vi "_TangoExtractArchivedData.vi"(2 "error in":errorcluster, 3 "db_extractor_dev_name":string, 4 "sampling":string, 5 "to_date":string, 6 "from_date":string, 7 "archived_attr_name":string) -> (0 "error out":errorcluster, 1 "attr values":T1(array[cluster]))   [LabVIEW 2014, in "tango.lvlib"]
uses:
  tango.lvlib
  Private VIs/Commands/Insertors/fromDevVarStringArray.vi
  Private VIs/Commands/Extractors/toDevVarLongStringArray.vi
  Private VIs/Commands/Insertors/fromDevString.vi
  tango_binding.so
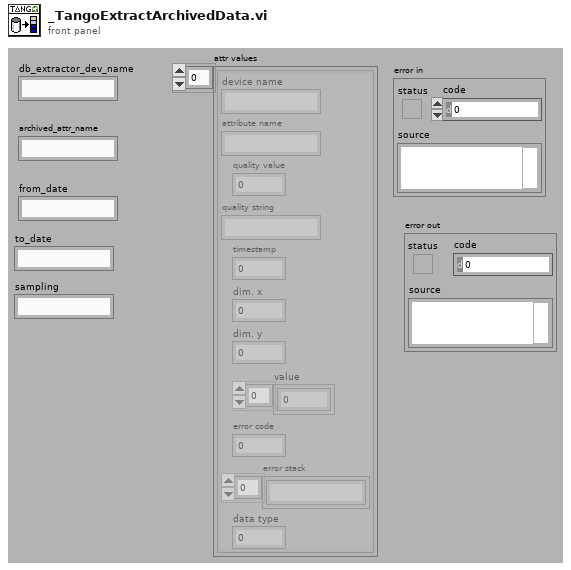
[diagram p1: front panel]
types:
  T1 = cluster{"device name":string, "attribute name":string, "quality value":i16, "quality string":string, "timestamp":dbl, "dim. x":i32, "dim. y":i32, "value":u8[], "error code":i32, "error stack":string[], "data type":u16}[]
  T2 = cluster{"device name":string, "attribute name":string, "quality value":i16, "quality string":string, "timestamp":dbl, "dim. x":i32, "dim. y":i32, "value":u8[], "error code":i32, "error stack":string[], "data type":u16}
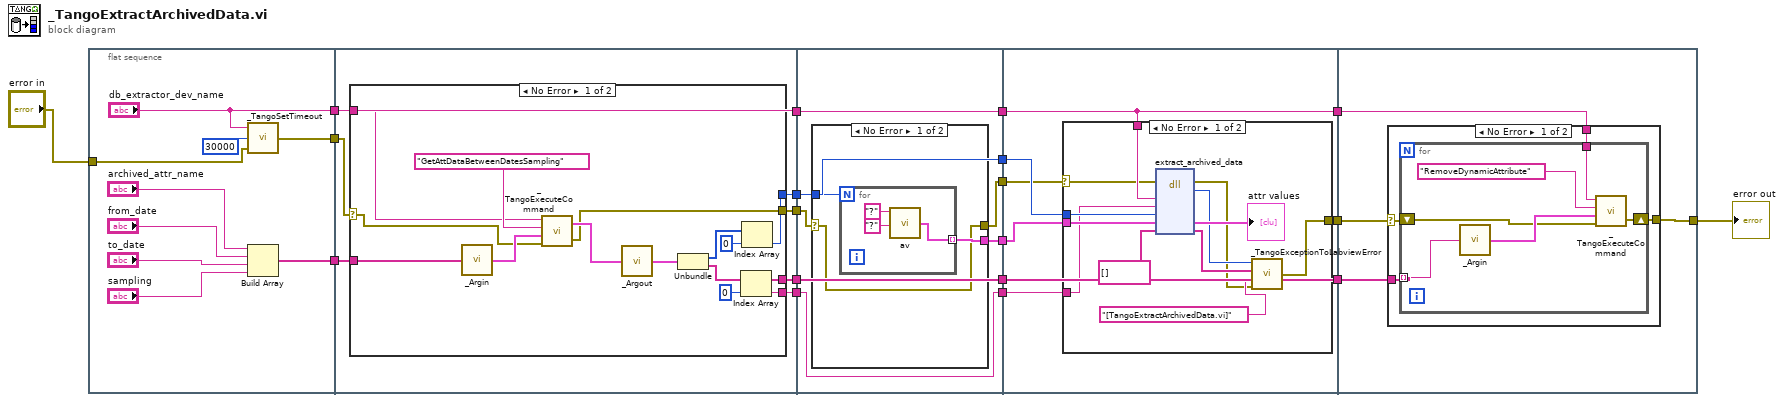
[diagram p0: block diagram]
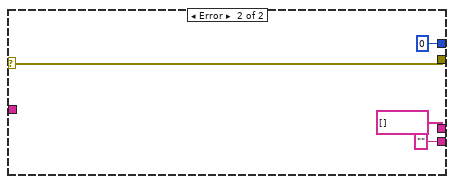
[diagram p2: hidden frame]
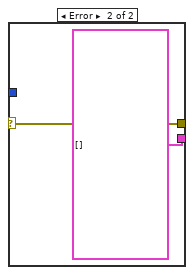
[diagram p3: hidden frame]
diagram:
  n1 = flat-sequence {
    tunnel: ["db_extractor_dev_name"] -> w19
    tunnel: [w24] -> w18
    tunnel: [w21] -> w9
    tunnel: "error in" -> [w20]
    tunnel: w19 -> [w33]
    tunnel: w18 -> [w35]
    tunnel: [w34] -> w17
    tunnel: [w33] -> w14
    tunnel: [w32] -> w12
    tunnel: w9 -> [w31]
    tunnel: [w30] -> w8
    tunnel: [w29] -> w2
    tunnel: w17 -> [w58]
    tunnel: [w60] -> w16
    tunnel: [w59] -> w15
    tunnel: w14 -> [w59]
    tunnel: [w55] -> w13
    tunnel: w12 -> [w55]
    tunnel: [w58] -> w11
    tunnel: w8 -> [w57]
    tunnel: [w56] -> w7
    tunnel: [w54] -> w3
    tunnel: w2 -> [w54]
    tunnel: w16 -> [w75]
    tunnel: w15 -> [w72]
    tunnel: w13 -> [w73]
    tunnel: w11 -> [w74]
    tunnel: [w72] -> w10
    tunnel: w7 -> [w70]
    tunnel: [w71] -> w6
    tunnel: [w69] -> w4
    tunnel: w3 -> [w69]
    tunnel: w10 -> [w92]
    tunnel: w6 -> [w91]
    tunnel: [w90] -> w1
    tunnel: w4 -> [w89]
    frame #0 {
      n2 = call "_TangoSetTimeout.vi"("error in"=w20, "tmo_in_msecs"=u32 30000, "device_name"="db_extractor_dev_name") -> ("error out"=w21:errorcluster)
      n3 = Build Array("archived_attr_name", "from_date", "to_date", "sampling") -> (w24:string[])
    }
    frame #1 {
      n4 = case shown="No Error" w31 {
        selector: w31 -> [w38 w53]
        tunnel: w35 -> [w45 _]
        tunnel: [w41 0] -> w34
        tunnel: w33 -> [w40 _]
        tunnel: [w39 ""] -> w32
        tunnel: [w37 w53] -> w30
        tunnel: [w36 string[] [] ("svalue")] -> w29
        frame No Error {
          n5 = call-poly "_Argin.vi"("argin"=w45) -> ("ArgIO"=w47:cluster{"num data":u8[], "str data":string[]})
          n6 = call "_TangoExecuteCommand.vi"("error in"=w38, "argin"=w47, "command name"="GetAttDataBetweenDatesSampling", "device name"=w40) -> ("error out"=w37:errorcluster, "argout"=w48:cluster{"num data":u8[], "str data":string[]})
          n7 = call-poly "_Argout.vi"("ArgIO"=w48) -> ("argout"=w49:cluster{"lvalue":i32[], "svalue":string[]})
          n8 = Unbundle(w49) -> ("lvalue"=w44:i32[], "svalue"=w36:string[])
          n9 = Index Array(array=w36, index=0) -> (element=w39:string)
          n10 = Index Array(array=w44, index=0) -> (element=w41:i32)
        }
        frame Error {
        }
      }
    }
    frame #2 {
      n11 = case shown="No Error" w57 {
        selector: w57 -> [w61 w68]
        tunnel: [w63 T1 []] -> w60
        tunnel: w58 -> [w62 _]
        tunnel: [w61 w68] -> w56
        frame No Error {
          n12 = for {
            N: w62 -> [_]
            tunnel: [w66] -> w63 mode=indexing
            n13 = call "av.vi"("attribute name"="?", "device name"="?") -> ("attribute value"=w66:T2)  [unwired: 4 in]
          }
        }
        frame Error {
        }
      }
    }
    frame #3 {
      n14 = case shown="No Error" w70 {
        selector: w70 -> [w76 w88]
        tunnel: w75 -> [w86 _]
        tunnel: w74 -> [w85 _]
        tunnel: w73 -> [w84 _]
        tunnel: w72 -> [w83 _]
        tunnel: [w77 w88] -> w71
        frame No Error {
          n15 = dll-call lib="tango_binding.*" fn="extract_archived_data"(error in=w76, "db_extractor_dev_name"=w83, "dynamic_attr_name"=w84, "dynamic_attr_history_len"=w85, "attr_values_inout"=w86, "error_stack"=string[] [] ("error stack")) -> (error out=w78:errorcluster, "return type"=w80:i32, "attr_values_inout"=→"attr values":T1, "error_stack"=w81:string[])  [unwired: 5 in, 1 out]
          n16 = call "_TangoExceptionToLabviewError.vi"("error in"=w78, "location"="[TangoExtractArchivedData.vi]", "error stack"=w81, "error code"=w80) -> ("error out"=w77:errorcluster)
        }
        frame Error {
        }
      }
    }
    frame #4 {
      n17 = case shown="No Error" w91 {
        selector: w91 -> [w94 w103]
        tunnel: w92 -> [w96 _]
        tunnel: [w95 w103] -> w90
        tunnel: w89 -> [w93 _]
        frame No Error {
          n18 = for {
            tunnel: w96 -> [w101]
            tunnel: w93 -> [w97] mode=indexing
            shift-right: [w99] -> w95
            shift-left: w94 -> [w98]
            n19 = call-poly "_Argin.vi"("argin"=w97) -> ("ArgIO"=w100:cluster{"num data":u8[], "str data":string[]})
            n20 = call "_TangoExecuteCommand.vi"("error in"=w98, "argin"=w100, "command name"="RemoveDynamicAttribute", "device name"=w101) -> ("error out"=w99:errorcluster)  [unwired: 1 out]
          }
        }
        frame Error {
        }
      }
    }
  }
  "error out" <- w1
